vi "get_digital_outputs_state.vi"(5 "Error In":errorcluster) -> (19 "Error Out":errorcluster)   [LabVIEW 2013, in "examples.lvlib"]
doc: "Produced By:\n\n<B>Kod Integrations, LLC</B>\n4835 Marianne Drive\nMount Airy, MD 21771\nhttp://www.kodintegrations.com\nemail: info@kodintegrations.com\nphone: (240) 687-1288"
uses:
  libraries/examples.lvlib
  classes/Controller/_Controller.lvclass
  common/controls/digital_output.ctl
  libraries/common.lvlib
  common/controls/digital_output_item.ctl
panel:
  out "do_items":T1[](array[typedef])
  out "dig_val (single only)":bool
  in  "get_all? (def=F)":bool
  in  "do (single)":T2
  in  "clear_buffer? (T)":bool=TRUE
  in  "device_index (in) [0=def]":i32
  # "instructions:\n\nThis VI can retrieve the status of ALL digital\noutput states or just that of a singale DO channel.\nIf retrieving ALL, set the input \"get_all?\" to TRUE \nand run the VI.\n\nIf retrieving just one, set the in put \"get_all?\" to\nFALSE (the default value) and select the digital\noutput channel value with the \"do (single)\" input\nand run the VI"
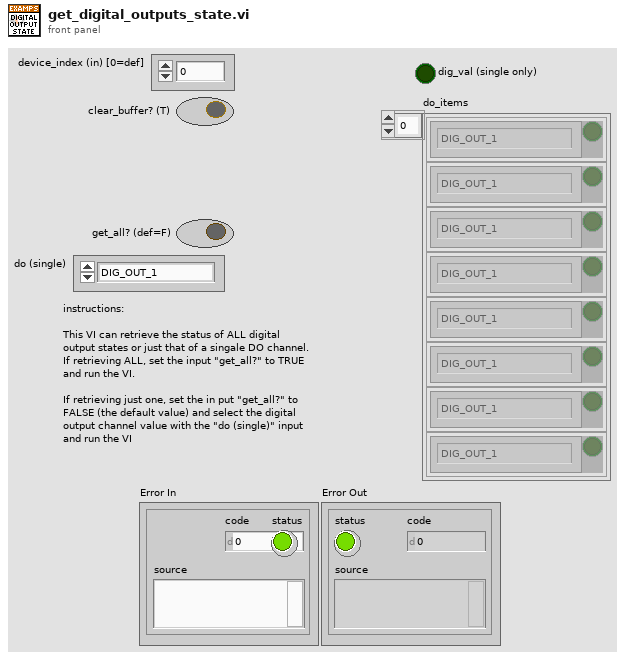
[diagram p1: front panel]
types:
  T1 = typedef "common.lvlib/digital_output_item.ctl" = cluster{"item":T2, "status":bool}
  T2 = typedef "common.lvlib/digital_output.ctl" = enum16{"DIG_OUT_1", "DIG_OUT_2", "DIG_OUT_3", "DIG_OUT_4", "DIG_OUT_5", "DIG_OUT_6", "DIG_OUT_7", "DIG_OUT_8"}
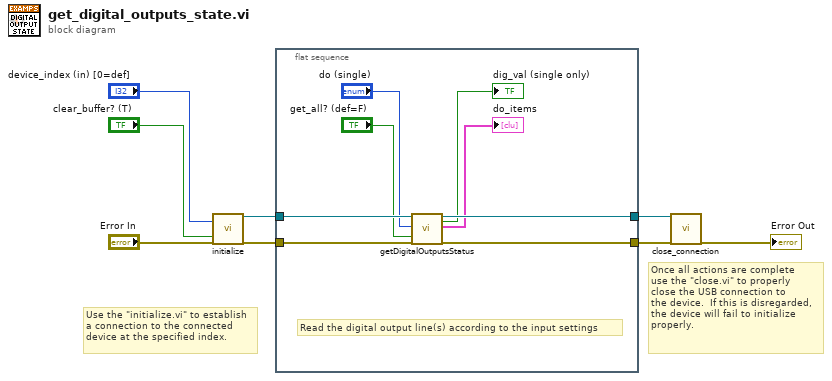
[diagram p0: block diagram]
diagram:
  # "Once all actions are complete\nuse the \"close.vi\" to properly\nclose the USB connection to \nthe device.  If this is disregarded,\nthe device will fail to initialize \nproperly."
  # "Use the \"initialize.vi\" to establish\na connection to the connected\ndevice at the specified index."
  n1 = call "initialize.vi"("device_index (in) [0=def]"="device_index (in) [0=def]", "clear_buffer? (T)"="clear_buffer? (T)", "error in (no error)"="Error In") -> ("reference (out)"=w5:refnum<class "_Controller.lvclass">, "error out"=w4:errorcluster)  [unwired: 15 in]
  n2 = flat-sequence {
    tunnel: w5 -> [w16]
    tunnel: w4 -> [w15]
    tunnel: [w14] -> w3
    tunnel: [w13] -> w2
    frame #0 {
      # "Read the digital output line(s) according to the input settings"
      n3 = call "getDigitalOutputsStatus.vi"("Controller in"=w16, "do (single)"="do (single)", "get_all? (def=F)"="get_all? (def=F)", "error in (no error)"=w15) -> ("Controller out"=w14:refnum<class "_Controller.lvclass">, "dig_val (single only)"=→"dig_val (single only)":bool, "do_items"=→"do_items":T1[], "error out"=w13:errorcluster)  [unwired: 11 in, 1 out]
    }
  }
  n4 = call "close_connection.vi"("reference (in)"=w3, "error in (no error)"=w2) -> ("error out"=→"Error Out":errorcluster)  [unwired: 16 in, 1 out]
